vi "Main.vi"(11 "error in (no error)":errorcluster) -> (15 "error out":errorcluster)   [LabVIEW 2020]
uses:
  Typedefs/Q_operation.ctl
  Typedefs/MainDataCluster.ctl
  Typedefs/TimeDetails.ctl
  Typedefs/Storage.ctl
  <vilib>/Utility/config.llb/Read Key (U32).vi
  <vilib>/Utility/config.llb/Read Key (Boolean).vi
  <vilib>/Utility/config.llb/Write Key (U32).vi
  <vilib>/Utility/config.llb/Write Key (String).vi
  <vilib>/Utility/config.llb/NI_LVConfig.lvlib
panel:
  in  "Power":bool
  out "Total Cups":u32
  out "Elapsed Time":u32
  out "Dispensing":bool
  out "Brewing":bool
  out "Grinding":bool
  out "Heating":bool
  out "Purging":bool
  out "Dispenser":dbl(slide) scale=0.0..60.0
  out "Chamber":dbl(slide) scale=0.0..60.0
  out "Low Milk":bool
  out "Low Bean":bool
  out "Low Water":bool
  in  "Milk Level":dbl(slide) scale=0.0..100.0
  in  "Bean Level":dbl(slide) scale=0.0..100.0
  in  "Water Level":dbl(slide) scale=0.0..100.0
  in  "Select Item":i32(knob) scale=0.0..2.0
  in  "1 Carafe":bool
  in  "1 Cup":bool
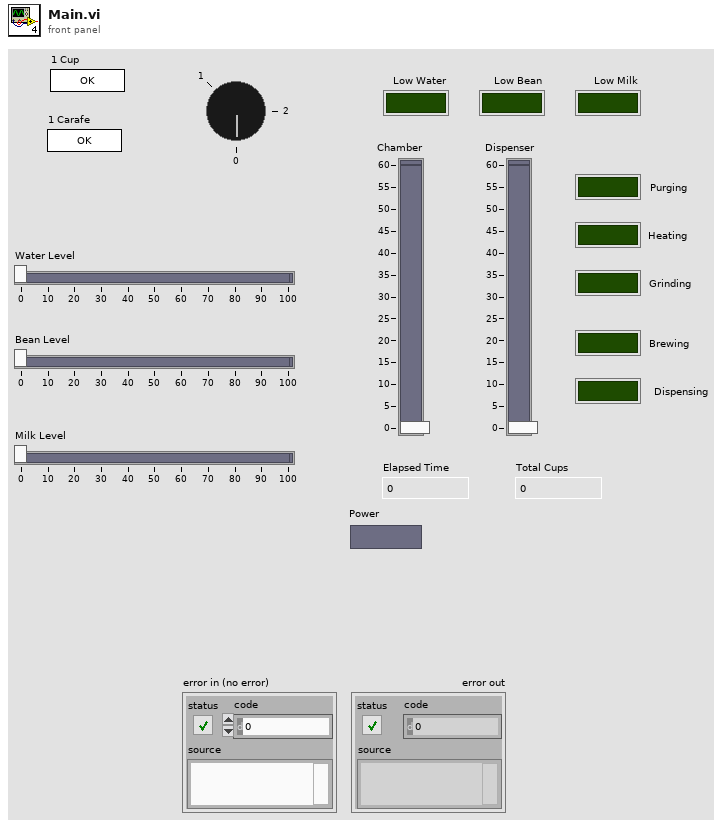
[diagram p1: front panel]
types:
  T1 = typedef "MainDataCluster.ctl" = cluster{"Low Milk":bool, "Low Water":bool, "Low Bean":bool, "Dispensing":bool, "Brewing":bool, "Grinding":bool, "Heating":bool, "Purging":bool, "Total Cups":u32, "TimeDetails":T2, "reference out":refnum<vi>, "Storage":T3, "Chamber":dbl, "Dispenser":dbl, "Path":path, "Enable":refnum<vi>[], "Disable":refnum<vi>[], "Shutdown?":bool, "Storage?":bool, "Secquence":string[], "Sequence Count":i32, "Selected Item":i32, "Cup/ Carafe":bool, "Shutdown Value":string}
  T2 = typedef "TimeDetails.ctl" = cluster{"Started":bool, "Paused":bool, "Stop":bool, "Elapsed Time":dbl, "Initial Time":dbl, "Set Time":dbl}
  T3 = typedef "Storage.ctl" = cluster{"Water Level":dbl, "Milk Level":dbl, "Bean Level":dbl}
  T4 = typedef "Q_operation.ctl" = enum16{"Create Q", "Enqueue 1", "Enqueue N", "Enstack 1", "Enstack N", "Dequeue", "Flush", "Release", "Preview"}
  T5 = enum8{"Enabled", "Disabled", "Disabled and Grayed Out"}
  T6 = typedef "NI_LVConfig.lvlib/Config Data RefNum.ctl" = refnum<k1>
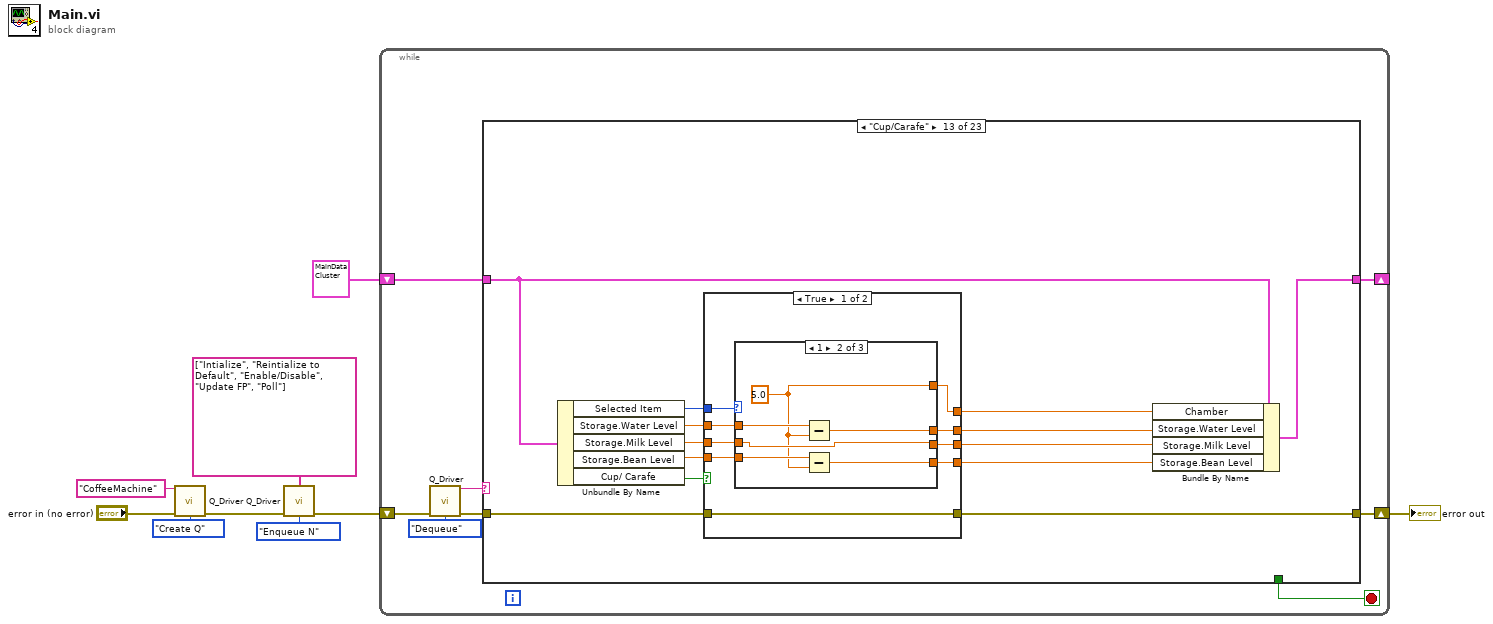
[diagram p0: block diagram]
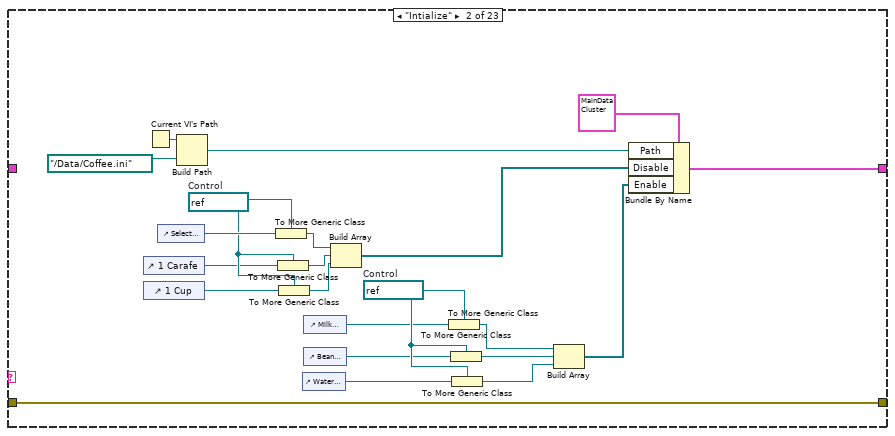
[diagram p3: hidden frame]
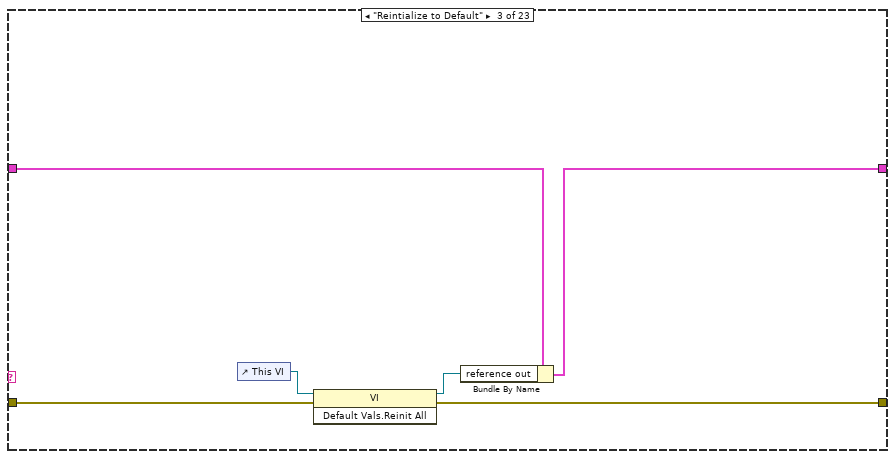
[diagram p4: hidden frame]
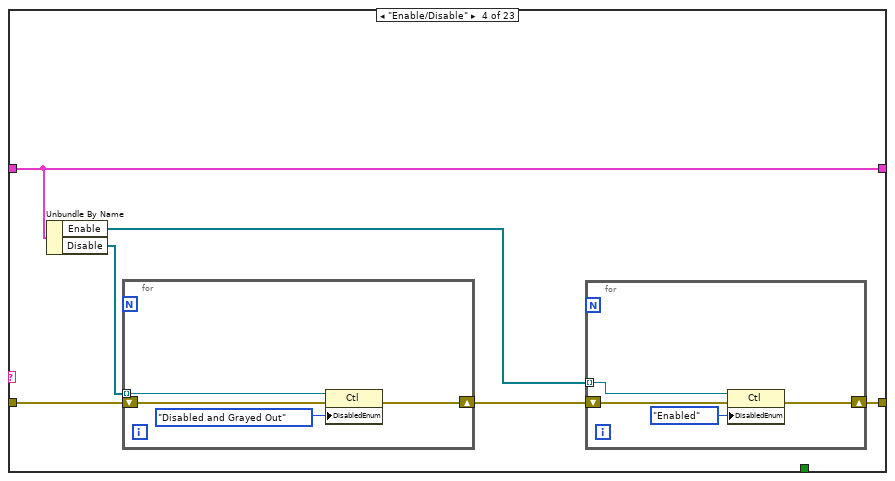
[diagram p5: hidden frame]
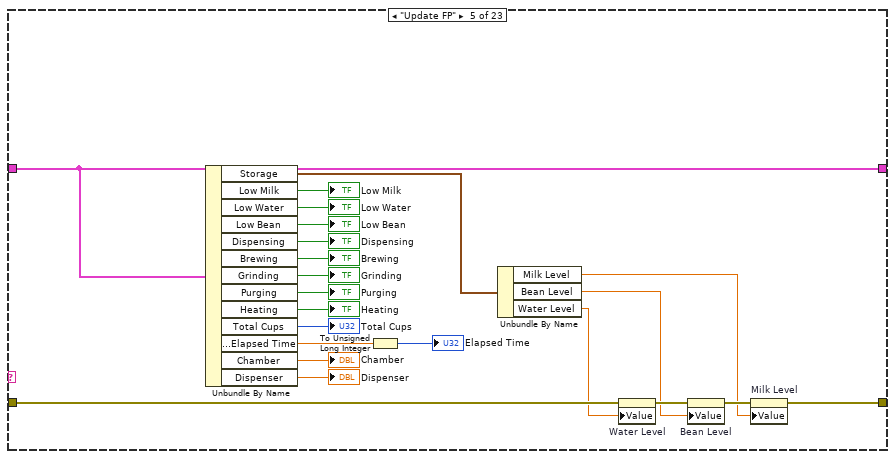
[diagram p6: hidden frame]
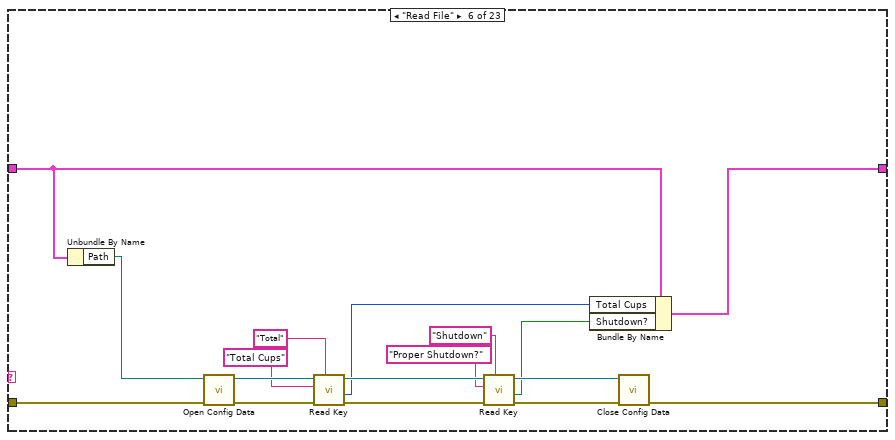
[diagram p7: hidden frame]
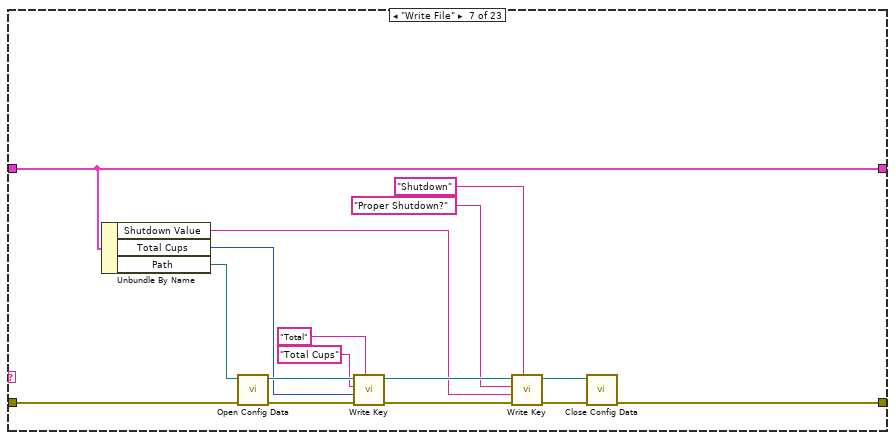
[diagram p8: hidden frame]
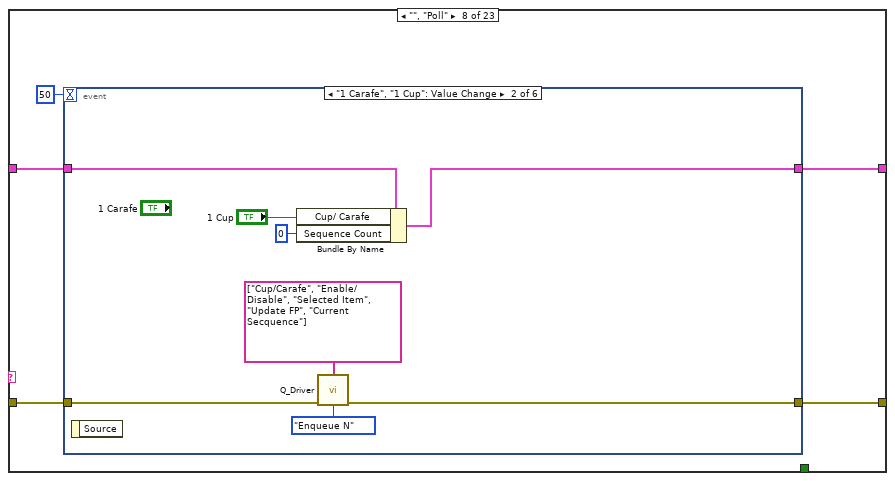
[diagram p9: hidden frame]
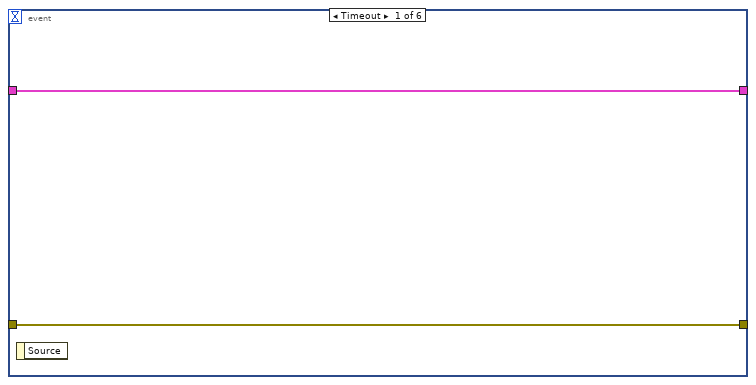
[diagram p10: hidden frame]
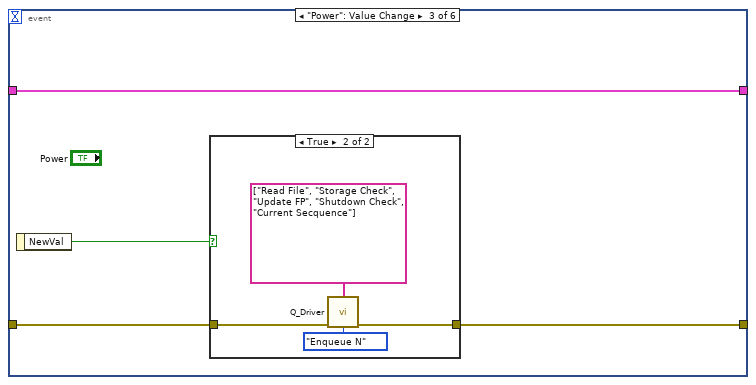
[diagram p11: hidden frame]
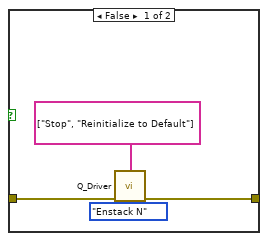
[diagram p12: hidden frame]
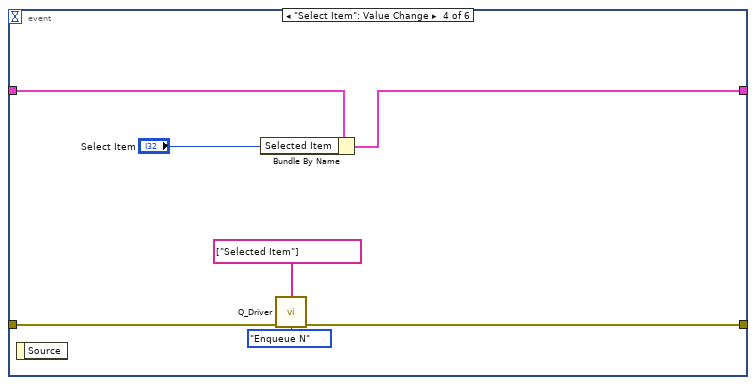
[diagram p13: hidden frame]
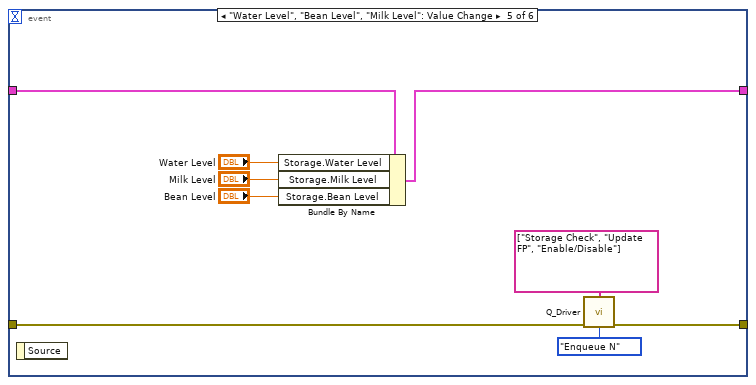
[diagram p14: hidden frame]
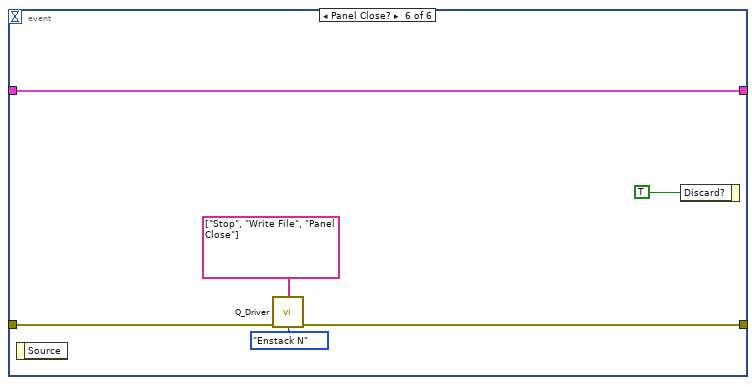
[diagram p15: hidden frame]
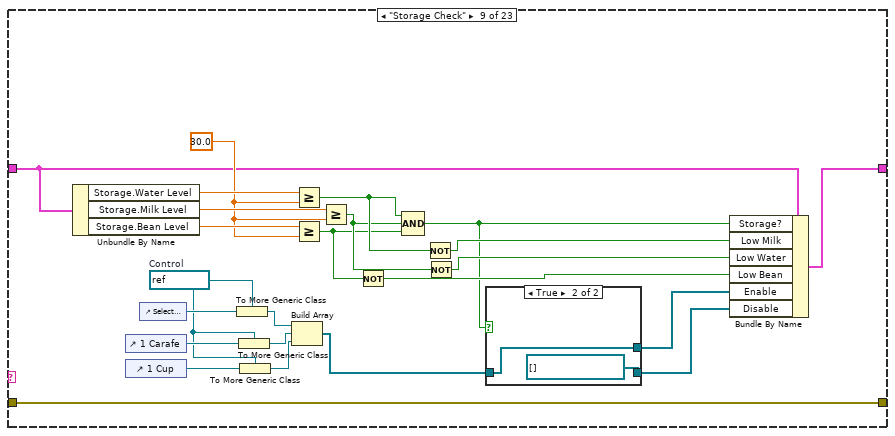
[diagram p16: hidden frame]
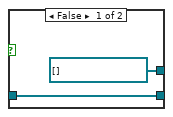
[diagram p17: hidden frame]
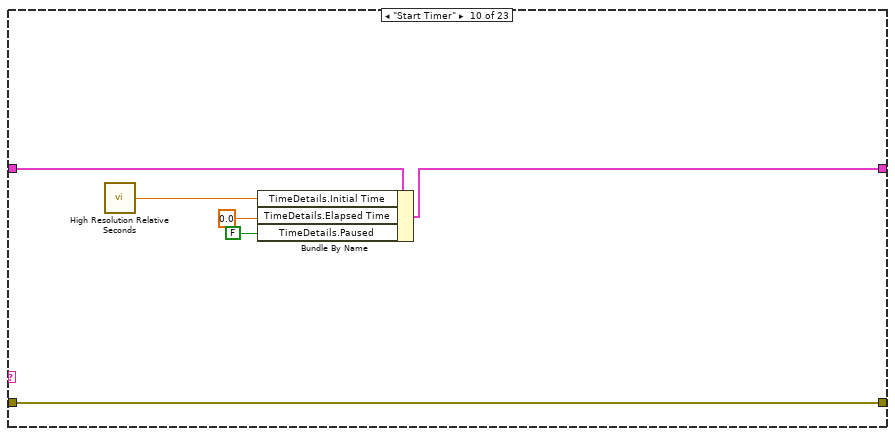
[diagram p18: hidden frame]
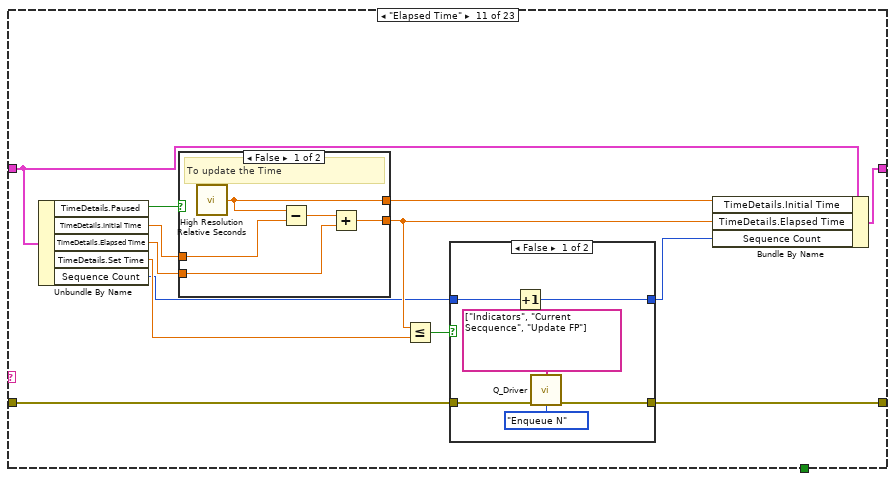
[diagram p19: hidden frame]
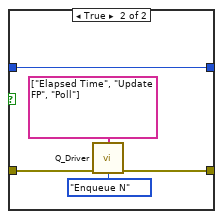
[diagram p20: hidden frame]
diagram:
  n1 = call "Q_Driver.vi"("Q_Name"="CoffeeMachine", "error in (no error)"="error in (no error)", "Q_Operation"=Q_operation."Create Q") -> ("error out"=w5:errorcluster)  [unwired: 10 in, 2 out]
  n2 = call "Q_Driver.vi"("States[]"=string[] ["Intialize", "Reintialize to Default", "Enable/Disable", "Update FP", "Poll"], "error in (no error)"=w5, "Q_Operation"=Q_operation."Enqueue N") -> ("error out"=w4:errorcluster)  [unwired: 10 in, 2 out]
  n3 = while {
    shift-right: [w17] -> w9
    shift-left: w4 -> [w16]
    shift-right: [w10] -> _
    shift-left: T1 {"Low Milk"=FALSE, "Low Water"=FALSE, "Low Bean"=FALSE, "Dispensing"=FALSE, "Brewing"=FALSE, "Grinding"=FALSE, "Heating"=FALSE, "Purging"=FALSE, "Total Cups"=0, "TimeDetails"={"Started"=FALSE, "Paused"=FALSE, "Stop"=FALSE, "Elapsed Time"=0.0, "Initial Time"=0.0, "Set Time"=0.0}, "reference out"=refnum, "Storage"={"Water Level"=0.0, "Milk Level"=0.0, "Bean Level"=0.0}, "Chamber"=0.0, "Dispenser"=0.0, "Path"=path "", "Enable"=[], "Disable"=[], "Shutdown?"=FALSE, "Storage?"=FALSE, "Secquence"=[], "Sequence Count"=0, "Selected Item"=0, "Cup/ Carafe"=FALSE, "Shutdown Value"=""} ("Cluster") -> [w11]
    stop <- w12 stop-if-true
    n4 = call "Q_Driver.vi"("error in (no error)"=w16, "Q_Operation"=Q_operation."Dequeue") -> ("State Out"=w13:string, "error out"=w15:errorcluster)  [unwired: 11 in, 1 out]
    n5 = case shown="\"Cup/Carafe\"" w13 {
      tunnel: [w19 w41 w47 w51 w67 w96 w109 w120 w177 w199 w203 w235 w242 w309 w339 w348 w376 w383 w392 w400 w410 w429 w432] -> w17
      tunnel: w15 -> [w19 w41 w46 w53 w66 w99 w115 w121 w177 w199 w204 w236 w243 w310 w339 w348 w375 w382 w391 w399 w409 w429 w437]
      tunnel: [_ _ _ _ _ _ _ _ _ _ _ _ _ _ _ _ _ _ _ _ _ _ TRUE] -> w12
      tunnel: w11 -> [w18 _ w44 w50 w71 w90 w116 w118 w184 w198 w209 w232 w251 w313 w337 w344 w378 w385 w388 w396 w406 w422 w430]
      tunnel: [w18 w37 w43 w50 w71 w91 w116 w117 w185 w197 w207 w233 w252 w313 w336 w343 w379 w386 w394 w402 w412 w423 w430] -> w10
      frame Default {
      }
      frame "Intialize" {
        w29 = refnum<vi> refnum  # Control
        w35 = refnum<vi> refnum  # Control
        n6 = control-ref of="1 Carafe"() -> (w34:refnum<vi>)
        n7 = control-ref of="1 Cup"() -> (w33:refnum<vi>)
        n8 = Current VI's Path() -> (path=w40:path)
        n9 = control-ref of="Select Item"() -> (w36:refnum<vi>)
        n10 = Build Path(base path=w40, name or relative path=path "../Data/Coffee.ini") -> (appended path=w38:path)
        n11 = To More Generic Class(target class=w35, reference=w36) -> (generic class reference=w32:refnum<vi>)
        n12 = To More Generic Class(target class=w35, reference=w34) -> (generic class reference=w31:refnum<vi>)
        n13 = To More Generic Class(target class=w35, reference=w33) -> (generic class reference=w30:refnum<vi>)
        n14 = control-ref of="Water Level"() -> (w26:refnum<vi>)
        n15 = control-ref of="Milk Level"() -> (w28:refnum<vi>)
        n16 = control-ref of="Bean Level"() -> (w27:refnum<vi>)
        n17 = Build Array(w32, w31, w30) -> (w22:refnum<vi>[])
        n18 = To More Generic Class(target class=w29, reference=w28) -> (generic class reference=w25:refnum<vi>)
        n19 = To More Generic Class(target class=w29, reference=w27) -> (generic class reference=w24:refnum<vi>)
        n20 = To More Generic Class(target class=w29, reference=w26) -> (generic class reference=w23:refnum<vi>)
        n21 = Build Array(w25, w24, w23) -> (w21:refnum<vi>[])
        n22 = Bundle By Name(cluster=T1 {"Low Milk"=FALSE, "Low Water"=FALSE, "Low Bean"=FALSE, "Dispensing"=FALSE, "Brewing"=FALSE, "Grinding"=FALSE, "Heating"=FALSE, "Purging"=FALSE, "Total Cups"=0, "TimeDetails"={"Started"=FALSE, "Paused"=FALSE, "Stop"=FALSE, "Elapsed Time"=0.0, "Initial Time"=0.0, "Set Time"=0.0}, "reference out"=refnum, "Storage"={"Water Level"=0.0, "Milk Level"=0.0, "Bean Level"=0.0}, "Chamber"=0.0, "Dispenser"=0.0, "Path"=path "", "Enable"=[], "Disable"=[], "Shutdown?"=FALSE, "Storage?"=FALSE, "Secquence"=[], "Sequence Count"=0, "Selected Item"=0, "Cup/ Carafe"=FALSE, "Shutdown Value"=""} ("Cluster"), "Path"=w38, "Disable"=w22, "Enable"=w21) -> (w37:T1)
      }
      frame "Reintialize to Default" {
        n23 = control-ref of="This VI"() -> (w45:refnum<vi>)
        n24 = invoke class="VI" method="Default Vals.Reinit All"(reference=w45, error in=w46) -> (reference out=w42:refnum<vi>, error out=w47:errorcluster)  [unwired: 1 in, 1 out]
        n25 = Bundle By Name(cluster=w44, "reference out"=w42) -> (w43:T1)
      }
      frame "Enable/Disable" {
        n26 = Unbundle By Name(w50) -> ("Enable"=w48:refnum<vi>[], "Disable"=w49:refnum<vi>[])
        n27 = for {
          shift-right: [w58] -> w52
          shift-left: w53 -> [w59]
          tunnel: w49 -> [w61] mode=indexing
          n28 = property class="Ctl"(reference=w61, error in=w59, "DisabledEnum"=T5."Disabled and Grayed Out" ("Disabled")) -> (error out=w58:errorcluster)  [unwired: 1 out]
        }
        n29 = for {
          shift-right: [w56] -> w51
          shift-left: w52 -> [w57]
          tunnel: w48 -> [w54] mode=indexing
          n30 = property class="Ctl"(reference=w54, error in=w57, "DisabledEnum"=T5."Enabled" ("Disabled")) -> (error out=w56:errorcluster)  [unwired: 1 out]
        }
      }
      frame "Update FP" {
        n31 = Unbundle By Name(w71) -> ("Storage"=w65:T3, "Low Milk"=→"Low Milk":bool, "Low Water"=→"Low Water":bool, "Low Bean"=→"Low Bean":bool, "Dispensing"=→"Dispensing":bool, "Brewing"=→"Brewing":bool, "Grinding"=→"Grinding":bool, "Purging"=→"Purging":bool, "Heating"=→"Heating":bool, "Total Cups"=→"Total Cups":u32, "TimeDetails.Elapsed Time"=w74:dbl, "Chamber"=→"Chamber":dbl, "Dispenser"=→"Dispenser":dbl)
        n32 = To Unsigned Long Integer(number=w74) -> (unsigned 32bit integer=→"Elapsed Time":u32)
        n33 = Unbundle By Name(w65) -> ("Milk Level"=w62:dbl, "Bean Level"=w63:dbl, "Water Level"=w64:dbl)
        n34 = property on="Water Level" class="Slide (strict)"(error in=w66, "Value"=w64) -> (error out=w69:errorcluster)  [unwired: 1 in, 1 out]
        n35 = property on="Bean Level" class="Slide (strict)"(error in=w69, "Value"=w63) -> (error out=w68:errorcluster)  [unwired: 1 in, 1 out]
        n36 = property on="Milk Level" class="Slide (strict)"(error in=w68, "Value"=w62) -> (error out=w67:errorcluster)  [unwired: 1 in, 1 out]
      }
      frame "Read File" {
        n37 = Unbundle By Name(w90) -> ("Path"=w100:path)
        n38 = call <vilib>:"Open Config Data.vi"("error in (no error)"=w99, "configuration file path"=w100) -> ("error out"=w97:errorcluster, "refnum"=w98:T6)  [unwired: 7 in, 1 out]
        n39 = call-poly <vilib>:"Read Key.vi"("section"="Total", "error in (no error)"=w97, "key"="Total Cups" ("section"), "refnum"=w98) -> ("error out"=w95:errorcluster, "value"=w89:u32, "refnum out"=w93:T6)  [unwired: 4 in, 1 out]
        n40 = call-poly <vilib>:"Read Key.vi"("section"="Shutdown", "error in (no error)"=w95, "key"="Proper Shutdown?" ("section"), "refnum"=w93) -> ("error out"=w94:errorcluster, "value"=w84:bool, "refnum out"=w92:T6)  [unwired: 4 in, 1 out]
        n41 = Bundle By Name(cluster=w90, "Total Cups"=w89, "Shutdown?"=w84) -> (w91:T1)
        n42 = call <vilib>:"Close Config Data.vi"("error in (no error)"=w94, "refnum"=w92) -> ("error out"=w96:errorcluster)  [unwired: 8 in, 1 out]
      }
      frame "Write File" {
        n43 = Unbundle By Name(w116) -> ("Shutdown Value"=w101:string, "Total Cups"=w110:u32, "Path"=w114:path)
        n44 = call <vilib>:"Open Config Data.vi"("error in (no error)"=w115, "configuration file path"=w114) -> ("error out"=w113:errorcluster, "refnum"=w112:T6)  [unwired: 7 in, 1 out]
        n45 = call-poly <vilib>:"Write Key.vi"("section"="Total", "error in (no error)"=w113, "value"=w110, "key"="Total Cups", "refnum"=w112) -> ("error out"=w105:errorcluster, "refnum out"=w107:T6)  [unwired: 4 in, 1 out]
        n46 = call-poly <vilib>:"Write Key.vi"("section"="Shutdown", "error in (no error)"=w105, "value"=w101, "key"="Proper Shutdown?" ("section"), "refnum"=w107) -> ("error out"=w104:errorcluster, "refnum out"=w106:T6)  [unwired: 4 in, 1 out]
        n47 = call <vilib>:"Close Config Data.vi"("error in (no error)"=w104, "refnum"=w106) -> ("error out"=w109:errorcluster)  [unwired: 8 in, 1 out]
      }
      frame "", "Poll" {
        n48 = event shown="[1] \"1 Carafe\", \"1 Cup\": Value Change" {
          selector: _ -> [_ _ _ _ _ _]
          dyn-events: _ -> [_ _ _ _ _ _]
          timeout: 50 -> [_ _ _ _ _ _]
          tunnel: [w123 w131 w134 w148 w154 w163] -> w120
          tunnel: w121 -> [w123 w130 w133 w147 w153 w164]
          tunnel: w118 -> [w122 w127 w135 w150 w158 w160]
          tunnel: [w122 w128 w135 w149 w159 w160] -> w117
          event Timeout {
            n49 = event-data() -> ()  [unwired: 1 in, 1 out]
          }
          event "1 Carafe", "1 Cup": Value Change {
            n50 = event-data() -> ()  [unwired: 1 in, 1 out]
            n51 = Bundle By Name(cluster=w127, "Cup/ Carafe"="1 Cup", "Sequence Count"=0) -> (w128:T1)
            n52 = call "Q_Driver.vi"("States[]"=string[] ["Cup/Carafe", "Enable/Disable", "Selected Item", "Update FP", "Current Secquence"], "error in (no error)"=w130, "Q_Operation"=Q_operation."Enqueue N") -> ("error out"=w131:errorcluster)  [unwired: 10 in, 2 out]
          }
          event "Power": Value Change {
            n53 = event-data() -> ("NewVal"=w132:bool)  [unwired: 1 in]
            n54 = case shown="True" w132 {
              tunnel: [w139 w143] -> w134
              tunnel: w133 -> [w138 w142]
              frame False {
                n55 = call "Q_Driver.vi"("States[]"=string[] ["Stop", "Reinitialize to Default"], "error in (no error)"=w138, "Q_Operation"=Q_operation."Enstack N") -> ("error out"=w139:errorcluster)  [unwired: 10 in, 2 out]
              }
              frame True {
                n56 = call "Q_Driver.vi"("States[]"=string[] ["Read File", "Storage Check", "Update FP", "Shutdown Check", "Current Secquence"], "error in (no error)"=w142, "Q_Operation"=Q_operation."Enqueue N") -> ("error out"=w143:errorcluster)  [unwired: 10 in, 2 out]
              }
            }
          }
          event "Select Item": Value Change {
            n57 = event-data() -> ()  [unwired: 1 in, 1 out]
            n58 = Bundle By Name(cluster=w150, "Selected Item"="Select Item") -> (w149:T1)
            n59 = call "Q_Driver.vi"("States[]"=string[] ["Selected Item"], "error in (no error)"=w147, "Q_Operation"=Q_operation."Enqueue N") -> ("error out"=w148:errorcluster)  [unwired: 10 in, 2 out]
          }
          event "Water Level", "Bean Level", "Milk Level": Value Change {
            n60 = event-data() -> ()  [unwired: 1 in, 1 out]
            n61 = Bundle By Name(cluster=w158, "Storage.Water Level"="Water Level", "Storage.Milk Level"="Milk Level", "Storage.Bean Level"="Bean Level") -> (w159:T1)
            n62 = call "Q_Driver.vi"("States[]"=string[] ["Storage Check", "Update FP", "Enable/Disable"], "error in (no error)"=w153, "Q_Operation"=Q_operation."Enqueue N") -> ("error out"=w154:errorcluster)  [unwired: 10 in, 2 out]
          }
          event Panel Close? {
            n63 = event-data() -> ()  [unwired: 1 in, 1 out]
            n64 = call "Q_Driver.vi"("States[]"=string[] ["Stop", "Write File", "Panel Close"], "error in (no error)"=w164, "Q_Operation"=Q_operation."Enstack N") -> ("error out"=w163:errorcluster)  [unwired: 10 in, 2 out]
            n65 = event-data("Discard?"=TRUE) -> ()  [unwired: 1 in, 1 out]
          }
        }
      }
      frame "Storage Check" {
        w170 = refnum<vi> refnum  # Control
        w186 = 30.0 ("y")
        n66 = Unbundle By Name(w184) -> ("Storage.Water Level"=w189:dbl, "Storage.Milk Level"=w188:dbl, "Storage.Bean Level"=w187:dbl)
        n67 = control-ref of="1 Carafe"() -> (w174:refnum<vi>)
        n68 = control-ref of="1 Cup"() -> (w173:refnum<vi>)
        n69 = control-ref of="Select Item"() -> (w175:refnum<vi>)
        n70 = To More Generic Class(target class=w170, reference=w175) -> (generic class reference=w172:refnum<vi>)
        n71 = To More Generic Class(target class=w170, reference=w174) -> (generic class reference=w171:refnum<vi>)
        n72 = To More Generic Class(target class=w170, reference=w173) -> (generic class reference=w169:refnum<vi>)
        n73 = Build Array(w172, w171, w169) -> (w168:refnum<vi>[])
        n74 = Greater Or Equal?(x=w189, y=w186) -> (x >= y?=w183:bool)
        n75 = Greater Or Equal?(x=w187, y=w186) -> (x >= y?=w178:bool)
        n76 = Greater Or Equal?(x=w188, y=w186) -> (x >= y?=w179:bool)
        n77 = Not(x=w178) -> (.not. x?=w180:bool)
        n78 = Compound Arithmetic op=AND(w183, w179, w178) -> (w176:bool)
        n79 = Not(x=w183) -> (.not. x?=w182:bool)
        n80 = Not(x=w179) -> (.not. x?=w181:bool)
        n81 = case shown="True" w176 {
          tunnel: w168 -> [w191 w193]
          tunnel: [refnum<vi>[] [] w193] -> w167
          tunnel: [w191 refnum<vi>[] []] -> w166
          frame False {
          }
          frame True {
          }
        }
        n82 = Bundle By Name(cluster=w184, "Storage?"=w176, "Low Milk"=w182, "Low Water"=w181, "Low Bean"=w180, "Enable"=w167, "Disable"=w166) -> (w185:T1)
      }
      frame "Start Timer" {
        n83 = call <vilib>:"High Resolution Relative Seconds.vi"() -> ("relative seconds"=w196:dbl)
        n84 = Bundle By Name(cluster=w198, "TimeDetails.Initial Time"=w196, "TimeDetails.Elapsed Time"=0.0, "TimeDetails.Paused"=FALSE) -> (w197:T1)
      }
      frame "Elapsed Time" {
        n85 = Unbundle By Name(w209) -> ("TimeDetails.Paused"=w212:bool, "TimeDetails.Initial Time"=w211:dbl, "TimeDetails.Elapsed Time"=w210:dbl, "TimeDetails.Set Time"=w205:dbl, "Sequence Count"=w201:i32)
        n86 = case shown="False" w212 {
          tunnel: [w227 w229] -> w206
          tunnel: [w226 w230] -> w208
          tunnel: w211 -> [w225 w230]
          tunnel: w210 -> [w224 w229]
          frame False {
            # "To update the Time"
            n87 = call <vilib>:"High Resolution Relative Seconds.vi"() -> ("relative seconds"=w226:dbl)
            n88 = Subtract(x=w226, y=w225) -> (x-y=w228:dbl)
            n89 = Add(x=w228, y=w224) -> (x+y=w227:dbl)
          }
          frame True {
            # "To retaint the same time"
          }
        }
        n90 = Less Or Equal?(x=w206, y=w205) -> (x <= y?=w202:bool)
        n91 = case shown="False" w202 {
          tunnel: w204 -> [w217 w222]
          tunnel: [w218 w223] -> w203
          tunnel: w201 -> [w214 w219]
          tunnel: [w213 w219] -> w200
          frame False {
            n92 = Increment(x=w214) -> (x+1=w213:i32)
            n93 = call "Q_Driver.vi"("States[]"=string[] ["Indicators", "Current Secquence", "Update FP"], "error in (no error)"=w217, "Q_Operation"=Q_operation."Enqueue N") -> ("error out"=w218:errorcluster)  [unwired: 10 in, 2 out]
          }
          frame True {
            n94 = call "Q_Driver.vi"("States[]"=string[] ["Elapsed Time", "Update FP", "Poll"], "error in (no error)"=w222, "Q_Operation"=Q_operation."Enqueue N") -> ("error out"=w223:errorcluster)  [unwired: 10 in, 2 out]
          }
        }
        n95 = Bundle By Name(cluster=w209, "TimeDetails.Initial Time"=w208, "TimeDetails.Elapsed Time"=w206, "Sequence Count"=w200) -> (w207:T1)
      }
      frame "Shutdown Check" {
        n96 = Unbundle By Name(w232) -> ("Shutdown?"=w234:bool)
        n97 = case shown="True" w234 {
          tunnel: w236 -> [w237 w240]
          tunnel: [w237 w240] -> w235
          tunnel: [string[] ["Purging", "Heating"] ("Power On Secquence") string[] ["Heating"] ("Power On Secquence")] -> w231
          frame False {
          }
          frame True {
          }
        }
        n98 = Bundle By Name(cluster=w232, "Secquence"=w231) -> (w233:T1)
      }
      frame "Cup/Carafe" {
        n99 = Unbundle By Name(w251) -> ("Selected Item"=w247:i32, "Storage.Water Level"=w250:dbl, "Storage.Milk Level"=w249:dbl, "Storage.Bean Level"=w248:dbl, "Cup/ Carafe"=w253:bool)
        n100 = case shown="True" w253 {
          tunnel: w250 -> [w261 w288]
          tunnel: w249 -> [w257 w284]
          tunnel: w248 -> [w259 w286]
          tunnel: w247 -> [w262 w289]
          tunnel: [w260 w287] -> w246
          tunnel: [w258 w285] -> w245
          tunnel: [w256 w283] -> w244
          tunnel: w243 -> [w255 w282]
          tunnel: [w255 w282] -> w242
          tunnel: [w254 w281] -> w241
          frame True {
            n101 = case shown="1" w262 {
              tunnel: w261 -> [w267 w273 w280]
              tunnel: [w266 w271 w277] -> w260
              tunnel: w259 -> [w264 w272 w279]
              tunnel: [w264 w270 w276] -> w258
              tunnel: w257 -> [w265 w269 w278]
              tunnel: [w265 w269 w275] -> w256
              tunnel: [w263 w268 w274] -> w254
              frame 0, Default {
                w263 = 5.0 ("y")
                n102 = Subtract(x=w267, y=w263) -> (x-y=w266:dbl)
              }
              frame 1 {
                w268 = 5.0 ("y")
                n103 = Subtract(x=w273, y=w268) -> (x-y=w271:dbl)
                n104 = Subtract(x=w272, y=w268) -> (x-y=w270:dbl)
              }
              frame 2 {
                w274 = 5.0 ("y")
                n105 = Subtract(x=w280, y=w274) -> (x-y=w277:dbl)
                n106 = Subtract(x=w278, y=w274) -> (x-y=w275:dbl)
                n107 = Subtract(x=w279, y=w274) -> (x-y=w276:dbl)
              }
            }
          }
          frame False {
            n108 = case shown="2" w289 {
              tunnel: w288 -> [w294 w300 w307]
              tunnel: [w293 w298 w304] -> w287
              tunnel: w286 -> [w291 w299 w306]
              tunnel: [w291 w297 w303] -> w285
              tunnel: w284 -> [w292 w296 w305]
              tunnel: [w292 w296 w302] -> w283
              tunnel: [w290 w295 w301] -> w281
              frame 0, Default {
                w290 = 20.0 ("y")
                n109 = Subtract(x=w294, y=w290) -> (x-y=w293:dbl)
              }
              frame 1 {
                w295 = 20.0 ("y")
                n110 = Subtract(x=w300, y=w295) -> (x-y=w298:dbl)
                n111 = Subtract(x=w299, y=w295) -> (x-y=w297:dbl)
              }
              frame 2 {
                w301 = 20.0 ("y")
                n112 = Subtract(x=w307, y=w301) -> (x-y=w304:dbl)
                n113 = Subtract(x=w305, y=w301) -> (x-y=w302:dbl)
                n114 = Subtract(x=w306, y=w301) -> (x-y=w303:dbl)
              }
            }
          }
        }
        n115 = Bundle By Name(cluster=w251, "Chamber"=w241, "Storage.Water Level"=w246, "Storage.Milk Level"=w244, "Storage.Bean Level"=w245) -> (w252:T1)
      }
      frame "Current Secquence" {
        n116 = Unbundle By Name(w313) -> ("Secquence"=w312:string[], "Sequence Count"=w311:i32)
        n117 = Index Array(array=w312, index=w311) -> (element=w308:string)
        n118 = case shown="\"Grinding\"" w308 {
          selector: w308 -> [w314 w318 w322 w326 w330 _]
          tunnel: w310 -> [w316 w320 w324 w328 w332 w334]
          tunnel: [w317 w321 w325 w329 w333 w334] -> w309
          frame "Heating" {
            n119 = call "Q_Driver.vi"("State"=w314, "error in (no error)"=w316, "Q_Operation"=Q_operation."Enqueue 1") -> ("error out"=w317:errorcluster)  [unwired: 10 in, 2 out]
          }
          frame "Purging" {
            n120 = call "Q_Driver.vi"("State"=w318, "error in (no error)"=w320, "Q_Operation"=Q_operation."Enqueue 1") -> ("error out"=w321:errorcluster)  [unwired: 10 in, 2 out]
          }
          frame "Dispensing" {
            n121 = call "Q_Driver.vi"("State"=w322, "error in (no error)"=w324, "Q_Operation"=Q_operation."Enqueue 1") -> ("error out"=w325:errorcluster)  [unwired: 10 in, 2 out]
          }
          frame "Brewing" {
            n122 = call "Q_Driver.vi"("State"=w326, "error in (no error)"=w328, "Q_Operation"=Q_operation."Enqueue 1") -> ("error out"=w329:errorcluster)  [unwired: 10 in, 2 out]
          }
          frame "Grinding" {
            n123 = call "Q_Driver.vi"("State"=w330, "error in (no error)"=w332, "Q_Operation"=Q_operation."Enqueue 1") -> ("error out"=w333:errorcluster)  [unwired: 10 in, 2 out]
          }
          frame Default {
          }
        }
      }
      frame "Selected Item" {
        n124 = Unbundle By Name(w337) -> ("Selected Item"=w338:i32)
        n125 = case shown="0, Default" w338 {
          tunnel: [string[] ["Dispensing"] ("Secquence") string[] ["Grinding", "Brewing", "Dispensing"] ("Secquence") string[] ["Grinding", "Brewing", "Dispensing"] ("Secquence")] -> w335
          frame 0, Default {
          }
          frame 1 {
          }
          frame 2 {
          }
        }
        n126 = Bundle By Name(cluster=w337, "Secquence"=w335) -> (w336:T1)
      }
      frame "Indicators" {
        n127 = Unbundle By Name(w344) -> ("Secquence"=w347:string[], "Sequence Count"=w346:i32)
        n128 = Index Array(array=w347, index=w346) -> (element=w345:string)
        n129 = case shown="Default" w345 {
          tunnel: w344 -> [w352 w356 w360 w364 w368 w372]
          tunnel: [w351 w355 w359 w363 w365 w371] -> w343
          frame "Purging" {
            w349 = FALSE ("Purging")
            n130 = Bundle By Name(cluster=w352, "Purging"=TRUE, "Heating"=w349, "Grinding"=w349, "Brewing"=w349, "Dispensing"=w349) -> (w351:T1)
          }
          frame "Grinding" {
            w353 = FALSE ("Purging")
            n131 = Bundle By Name(cluster=w356, "Grinding"=TRUE ("Purging"), "Heating"=w353, "Purging"=w353, "Brewing"=w353, "Dispensing"=w353) -> (w355:T1)
          }
          frame "Brewing" {
            w357 = FALSE ("Purging")
            n132 = Bundle By Name(cluster=w360, "Brewing"=TRUE ("Purging"), "Heating"=w357, "Purging"=w357, "Grinding"=w357, "Dispensing"=w357) -> (w359:T1)
          }
          frame "Dispensing" {
            w361 = FALSE ("Purging")
            n133 = Bundle By Name(cluster=w364, "Dispensing"=TRUE ("Purging"), "Heating"=w361, "Purging"=w361, "Grinding"=w361, "Brewing"=w361) -> (w363:T1)
          }
          frame "Heating" {
            w366 = FALSE ("Purging")
            n134 = Bundle By Name(cluster=w368, "Heating"=TRUE, "Purging"=w366, "Grinding"=w366, "Brewing"=w366, "Dispensing"=w366) -> (w365:T1)
          }
          frame Default {
            w370 = FALSE ("Dispensing")
            n135 = Bundle By Name(cluster=w372, "Dispensing"=w370, "Brewing"=w370, "Grinding"=w370, "Heating"=w370, "Purging"=w370, "TimeDetails.Elapsed Time"=0.0) -> (w371:T1)
          }
        }
      }
      frame "Heating" {
        n136 = call "Q_Driver.vi"("States[]"=string[] ["Start Timer", "Indicators", "Elapsed Time"], "error in (no error)"=w375, "Q_Operation"=Q_operation."Enqueue N") -> ("error out"=w376:errorcluster)  [unwired: 10 in, 2 out]
        n137 = Bundle By Name(cluster=w378, "TimeDetails.Set Time"=5.0) -> (w379:T1)
      }
      frame "Purging" {
        n138 = call "Q_Driver.vi"("States[]"=string[] ["Start Timer", "Indicators", "Elapsed Time"], "error in (no error)"=w382, "Q_Operation"=Q_operation."Enqueue N") -> ("error out"=w383:errorcluster)  [unwired: 10 in, 2 out]
        n139 = Bundle By Name(cluster=w385, "TimeDetails.Set Time"=4.0) -> (w386:T1)
      }
      frame "Grinding" {
        n140 = Unbundle By Name(w388) -> ("Storage.Bean Level"=w387:dbl)
        n141 = Bundle By Name(cluster=w388, "TimeDetails.Set Time"=3.0, "Chamber"=w387) -> (w394:T1)
        n142 = call "Q_Driver.vi"("States[]"=string[] ["Start Timer", "Indicators", "Elapsed Time"], "error in (no error)"=w391, "Q_Operation"=Q_operation."Enqueue N") -> ("error out"=w392:errorcluster)  [unwired: 10 in, 2 out]
      }
      frame "Brewing" {
        n143 = Unbundle By Name(w396) -> ("Storage.Water Level"=w395:dbl)
        n144 = call "Q_Driver.vi"("States[]"=string[] ["Start Timer", "Indicators", "Elapsed Time"], "error in (no error)"=w399, "Q_Operation"=Q_operation."Enqueue N") -> ("error out"=w400:errorcluster)  [unwired: 10 in, 2 out]
        n145 = Bundle By Name(cluster=w396, "TimeDetails.Set Time"=4.0, "Chamber"=w395) -> (w402:T1)
      }
      frame "Dispensing" {
        n146 = Unbundle By Name(w406) -> ("Cup/ Carafe"=w405:bool, "Total Cups"=w404:u32)
        n147 = case shown="True" w405 {
          tunnel: w404 -> [w415 w417]
          tunnel: [w414 w416] -> w403
          frame False {
            n148 = Add(x=u32 4, y=w415) -> (x+y=w414:u32)
          }
          frame True {
            n149 = Increment(x=w417) -> (x+1=w416:u32)
          }
        }
        n150 = Bundle By Name(cluster=w406, "TimeDetails.Set Time"=5.0, "Total Cups"=w403) -> (w412:T1)
        n151 = call "Q_Driver.vi"("States[]"=string[] ["Start Timer", "Indicators", "Elapsed Time"], "error in (no error)"=w409, "Q_Operation"=Q_operation."Enqueue N") -> ("error out"=w410:errorcluster)  [unwired: 10 in, 2 out]
      }
      frame "Panel Close" {
        n152 = Unbundle By Name(w422) -> ("Brewing"=w428:bool, "Grinding"=w427:bool, "Heating"=w426:bool, "Purging"=w425:bool, "Dispensing"=w418:bool)
        n153 = Compound Arithmetic op=OR(w428, w427, w426, w425, w418) -> (w424:bool)
        n154 = Select(t="FALSE" ("Shutdown Value"), s=w424, f="TRUE" ("Shutdown Value")) -> (s? t:f=w420:string)
        n155 = Bundle By Name(cluster=w422, "Shutdown Value"=w420) -> (w423:T1)
      }
      frame "Stop" {
        n156 = call "Q_Driver.vi"("error in (no error)"=w437, "Q_Operation"=Q_operation."Flush") -> ("error out"=w435:errorcluster)  [unwired: 11 in, 2 out]
        n157 = call "Q_Driver.vi"("error in (no error)"=w435, "Q_Operation"=Q_operation."Release") -> ("error out"=w433:errorcluster)  [unwired: 11 in, 2 out]
        n158 = Unbundle By Name(w430) -> ("reference out"=w431:refnum<vi>)
        n159 = Close Reference(reference=w431, error in (no error)=w433) -> (error out=w432:errorcluster)
      }
    }
  }
  "error out" <- w9
